vi "AdjustOrientation.vi"(4 "orientation":dbl, 6 "target":dbl[](array[numeric]), 7 "initial pos":dbl[](array[numeric]), 8 "error in (no error)":errorcluster, 9 "dest":dbl[](array[numeric]), 10 "Game":refnum<class "Game.lvclass">, 11 "WaitBallTrajSkill in":refnum<class "WaitBallTrajSkill.lvclass">) -> (0 "error out":errorcluster, 1 "orientation out":dbl, 3 "WaitBallTrajSkill out":refnum<class "WaitBallTrajSkill.lvclass">)   [LabVIEW 2024, in "WaitBallTrajSkill.lvclass"]
uses:
  WaitBallTrajSkill.lvclass
  Game_class/Game.lvclass
  Game_class/Game.lvclass/Game.ctl
  <vilib>/Analysis/_algsub.llb/Real Vector Norm.vi
  Game_class/Read NewParameters.vi
  7f3eed74-8c84-4a47-a032-63cb7fcd0d91.vi
  Utilities_class/Utilities.lvclass
  <vilib>/Analysis/NI_AALPro.lvlib
  Robot_class/Robot.lvclass
  Ball_class/Ball.lvclass
  Field_class/Field.lvclass
panel:
  in  "MinDeviation at 80 degreees":dbl=0.46 format="%#_13g"
  in  "MinPassDistance":dbl=1000.0 format="%#_13g"
  in  "MaxPassDistance":dbl=4000.0 format="%#_13g"
  in  "MaxDeviation at 80 degrees":dbl=0.52 format="%#_13g"
  in  "Array":dbl[](array[numeric])
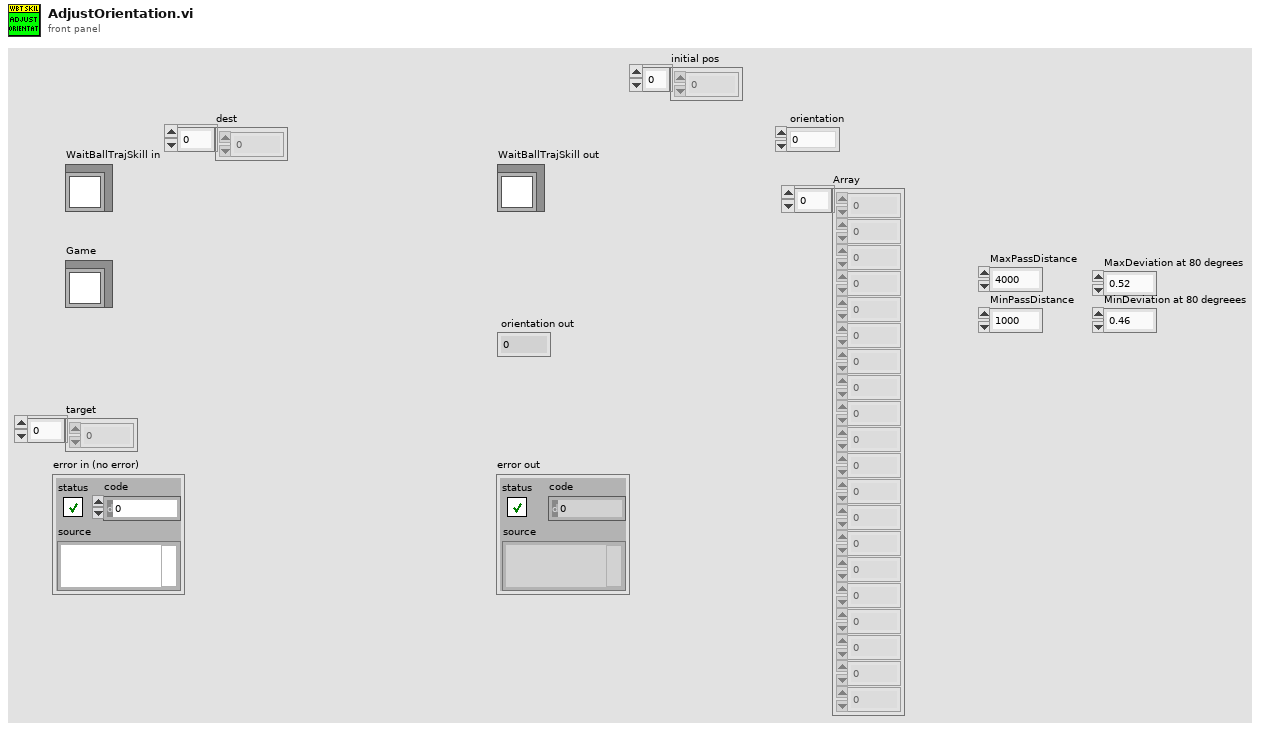
[diagram p1: front panel]
types:
  T1 = typedef "NewParameters.ctl" = cluster{"PenaltyDistance":dbl, "DistanceAttackerToBackBall":dbl, "Division":enum16{"Div B", "Div A"}, "DistanceToAvoidyEnemyRobot":dbl, "BallPlacementDistance":dbl, "DisatanceBehindBallToStealBall":dbl, "MaxDistanceToPositionKickoff":dbl, "BlockEnemyTarget":bool, "MaxStopVAng":dbl, "DistanceMarkerToEnemy":dbl, "IgnoreDribblerContact":bool, "DistanceToBeginEnemyPosession":dbl, "GoToBallWhenEnemyNotMoving":bool, "EnemyDistanceToReduceVelocity":dbl, "TurnOnEnemyDistanceToReduceVelocity":bool, "EnemyDistanceToShootOutBall":dbl, "DefenseKickBall":bool, "MoreKickToGoal? (0-0.3)":dbl, "ChipKickInEnemyField":bool, "ShootOutRobotId":dbl, "FieldLenghtDenominatorInShootOut":dbl, "AdjustPositionInBallPlacement":bool, "PowerGodPass":dbl, "VelocityAbortEnemyPos":dbl, "MaxDistToBeginPass":dbl, "MinDistToBeginPass":dbl, "VelocityInDirects":dbl, "BadDribblerIDs":i32[], "NewKickToDistanceAroundBall":dbl, "PowerAvoidColisionMarker":dbl, "DistanceToAvoidColisionMarker":dbl, "AvoidBallKick":dbl, "DistanceTryKick":dbl, "SuicideKickDIstance":dbl, "AdjustFirstKickDistance":dbl, "AvoidAimLessKick":dbl, "DistanceToAvoidyEnemyShootRobot ":dbl, "NumberOfMarkers":dbl, "PotField":bool, "PIDLateral":bool, "MinDistanceFirstKickX":dbl, "MinDistanceFirstKickY":dbl, "FractionOfDistToTouchGround\nAfterChipKick":dbl, "FractionOfKickxWhen\nComposedWithKickz":dbl, "Style":T2, "MoveInTurnState":bool, "DistFromEnemyToConsider\nMoveInTurnState":dbl, "CascadePID":bool, "TurnAroundParameters":cluster{"Radius":dbl, "Multiplier":dbl, "ChordAngle":dbl}, "SafeDriveVel":dbl, "DistanceToGoToBackBall":dbl, "minDistanceToNotFinish\nEnemyPossession":dbl, "OneTouchShot":cluster{"angleFactor":dbl, "maxAngle":dbl, "Attack":bool, "Defense":bool}, "OpenAngleToGoal":cluster{"minAngle":dbl, "maxAngle":dbl, "minEvaluation":dbl}, "ShotInterception":cluster{"shotSpeed":dbl, "minEnemySpeed":dbl, "maxEnemySpeed":dbl, "minEvaluation":dbl}, "AllyTeamArray":T3[], "maxDefendersNumber":i32, "Zone":cluster{"GuardPositionArray":dbl[][], "ZoneMidField":dbl[], "CenterForwardWidth":dbl}, "MinEvaluationToShoot":dbl, "PassInterception":cluster{"maxPassSpeed":dbl, "minPassSpeed":dbl, "minEnemySpeed":dbl, "chipPassDistance":dbl, "chipPassEvaluation":dbl, "minEvaluation":dbl, "maxEnemySpeed":dbl}, "PassDistance":cluster{"maxDistance":dbl, "minDistance":dbl}, "receiverSpeed":dbl, "maxBallSpeed":dbl, "slackTime":dbl, "Turning radius":dbl, "Turning v_ang":dbl, "AlignError":cluster{"Distance":dbl, "Orientation":dbl, "V_norm(m/s)":dbl, "V_ang (rad/s)":dbl}, "RobotRadius":dbl, "KickerDistance":dbl, "keeper angle  to cover goalpost":dbl, "a_slide":dbl, "a_roll":dbl, "k_switch":dbl}
  T2 = typedef "Style.ctl" = enum16{"Insanity", "Offensive", "Defensive"}
  T3 = typedef "AllyTeam.ctl" = enum16{"Keeper", "Defender", "Attacker"}
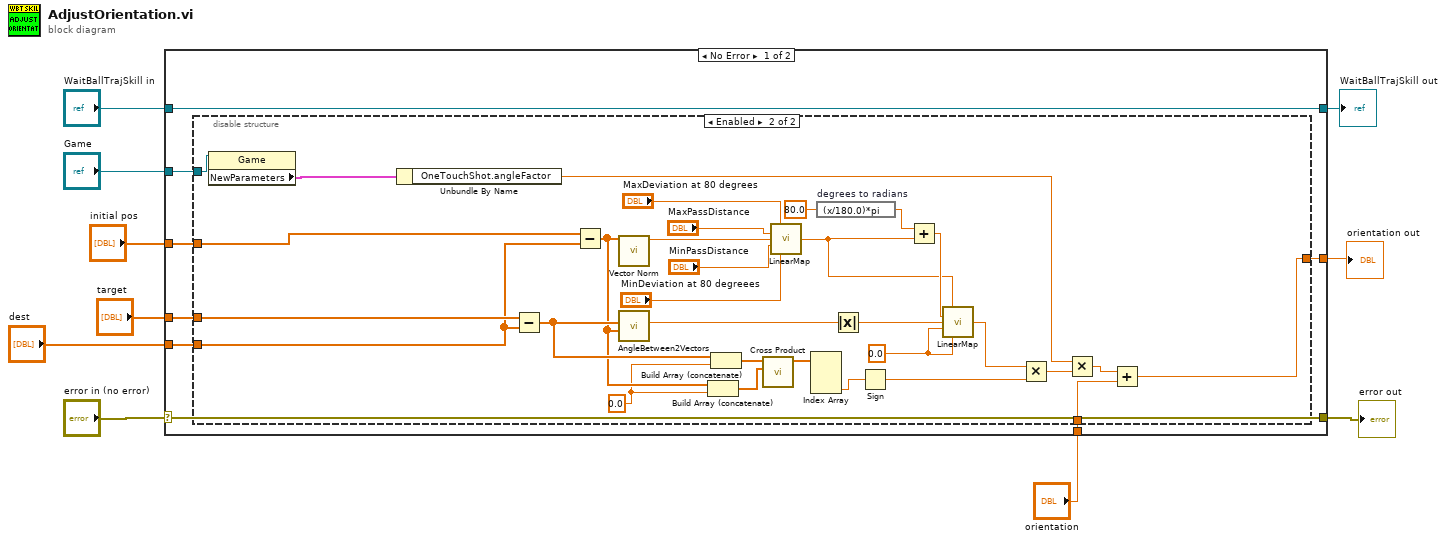
[diagram p0: block diagram]
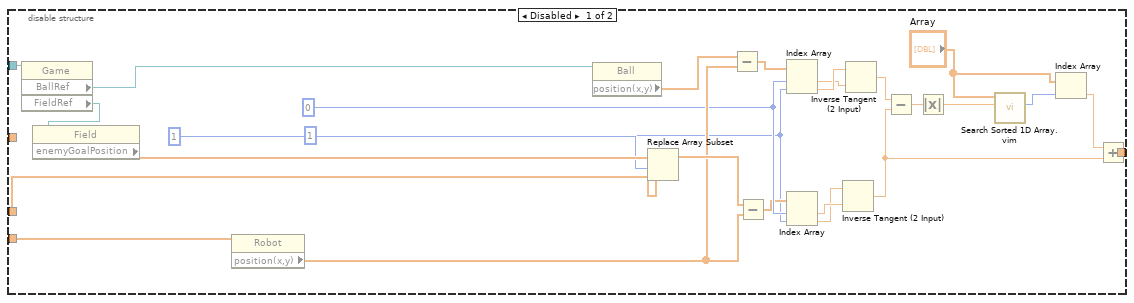
[diagram p2: hidden frame]
diagram:
  n1 = case shown="No Error" "error in (no error)" {
    selector: "error in (no error)" -> [w17 w77]
    tunnel: [w17 w77] -> w9
    tunnel: [w18 w76] -> w7
    tunnel: "WaitBallTrajSkill in" -> [w18 w76]
    tunnel: "Game" -> [w16 _]
    tunnel: "dest" -> [w15 _]
    tunnel: "target" -> [w14 _]
    tunnel: [w13 _] -> w4
    tunnel: "orientation" -> [w12 _]
    tunnel: "initial pos" -> [w11 _]
    frame No Error {
      n2 = disable-structure shown="Enabled" {
        disable-tunnel: w16 -> [w44 w69]
        disable-tunnel: w15 -> [w41 w66]
        disable-tunnel: w14 -> [w39 w67]
        disable-tunnel: [w21 w55] -> w13
        disable-tunnel: w12 -> [_ w56]
        disable-tunnel: w11 -> [_ w45]
        frame Disabled {
          w28 = 1
          w30 = 0
          n3 = property class="Game"(reference=w44) -> ("BallRef"=w43:refnum<class "Ball.lvclass">, "FieldRef"=w40:refnum<class "Field.lvclass">)  [unwired: 1 in, 2 out]
          n4 = property class="Field"(reference=w40) -> ("enemyGoalPosition"=w38:dbl[])  [unwired: 1 in, 2 out]
          n5 = property class="Robot"(reference=w41) -> ("position(x,y)"=w34:dbl[])  [unwired: 1 in, 2 out]
          n6 = property class="Ball"(reference=w43) -> ("position(x,y)"=w35:dbl[])  [unwired: 1 in, 2 out]
          n7 = Replace Array Subset(array=w38, new element=w39, index=1) -> (w36:dbl[])
          n8 = Subtract(x=w35, y=w34) -> (x-y=w31:dbl[])
          n9 = Subtract(x=w36, y=w34) -> (x-y=w29:dbl[])
          n10 = Index Array(array=w31, index #1=w30, index #2=w28) -> (element #1=w24:dbl, element #2=w25:dbl)
          n11 = Index Array(array=w29, index #1=w30, index #2=w28) -> (element #1=w27:dbl, element #2=w26:dbl)
          n12 = Inverse Tangent (2 Input)(1:w27, 2:w26) -> (0:w19:dbl)
          n13 = Inverse Tangent (2 Input)(1:w24, 2:w25) -> (0:w32:dbl)
          n14 = Subtract(x=w32, y=w19) -> (x-y=w42:dbl)
          n15 = Absolute Value(x=w42) -> (abs(x)=w33:dbl)
          n16 = call "Search Sorted 1D Array.vim"("element"=w33, "sorted 1D array"="Array") -> ("nearest index"=w22:i32)  [unwired: 8 in, 1 out]
          n17 = Index Array(array="Array", index=w22) -> (element=w20:dbl)
          n18 = Add(x=w20, y=w19) -> (x+y=w21:dbl)
        }
        frame Enabled {
          w51 = 0.0 ("element")
          w65 = 0.0 ("MinY")
          n19 = property class="Game"(reference=w69) -> ("NewParameters"=w47:T1)  [unwired: 1 in, 2 out]
          n20 = Unbundle By Name(w47) -> ("OneTouchShot.angleFactor"=w46:dbl)
          n21 = Subtract(x=w67, y=w66) -> (x-y=w54:dbl[])
          n22 = Subtract(x=w45, y=w66) -> (x-y=w52:dbl[])
          n23 = call-poly <vilib>:"Vector Norm.vi"("Input Vector"=w52) -> ("norm"=w68:dbl)  [unwired: 9 in, 1 out]
          n24 = call "AngleBetween2Vectors.vi"("Array 1"=w52, "Array 2"=w54) -> ("angleInRadians(default)"=w62:dbl)  [unwired: 6 in, 3 out]
          n25 = Build Array (concatenate)(w52, w51) -> (w50:dbl[])
          n26 = Build Array (concatenate)(w54, w51) -> (w53:dbl[])
          n27 = call <vilib>:"Cross Product.vi"("B Vector"=w50, "A Vector"=w53) -> ("Cross Product"=w58:dbl[])  [unwired: 8 in, 1 out]
          n28 = call "LinearMap.vi"("MaxY"="MaxDeviation at 80 degrees", "MaxX"="MaxPassDistance", "X"=w68, "MinX"="MinPassDistance", "MinY"="MinDeviation at 80 degreees") -> ("Y"=w63:dbl)  [unwired: 8 in, 2 out]
          n29 = Index Array(array=w58) -> (element #3=w57:dbl)  [unwired: 3 in, 2 out]
          n30 = expression code="(x/180.0)*pi" "degrees to radians"(80.0) -> (w70:dbl)
          n31 = Absolute Value(x=w62) -> (abs(x)=w61:dbl)
          n32 = Sign(1:w57) -> (0:w60:dbl)
          n33 = Add(x=w70, y=w63) -> (x+y=w64:dbl)
          n34 = call "LinearMap.vi"("MaxY"=w63, "MaxX"=w64, "X"=w61, "MinX"=w65, "MinY"=w65) -> ("Y"=w59:dbl)  [unwired: 8 in, 2 out]
          n35 = Multiply(x=w59, y=w60) -> (x*y=w49:dbl)
          n36 = Multiply(x=w46, y=w49) -> (x*y=w48:dbl)
          n37 = Add(x=w48, y=w56) -> (x+y=w55:dbl)
        }
      }
    }
    frame Error {
    }
  }
  "error out" <- w9
  "WaitBallTrajSkill out" <- w7
  "orientation out" <- w4
